vi "Write Alarms Event Response.vi"(8 "error in (no error)":errorcluster, 10 "Alarms":T1[](array[typedef]), 11 "Alarms in":refnum<class "HK Alarms.lvclass">) -> (0 "error out":errorcluster, 3 "Alarms out":refnum<class "HK Alarms.lvclass">)   [LabVIEW 2019, in "HK Alarms.lvclass"]
uses:
  HK Alarms/HK Alarms.lvclass
  HK Channel Settings Alarms.ctl
  HK Alarm enum Action.ctl
  HK Alarms/HK Alarms.lvclass/HK Alarms.ctl
  HK Item/HK Item.lvclass
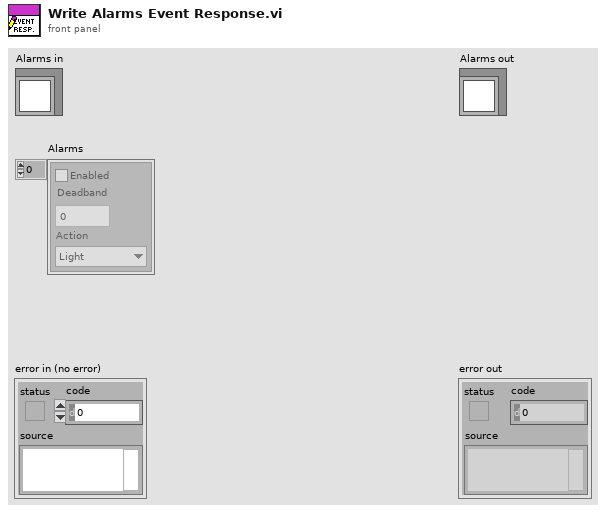
[diagram p1: front panel]
types:
  T1 = typedef "HK Item.lvclass/HK Channel Settings Alarms.ctl" = cluster{"Enabled":bool, "Deadband":i32, "Action":T2}
  T2 = typedef "HK Item.lvclass/HK Alarm enum Action.ctl" = enum16{"Light", "Message", "Safe"}
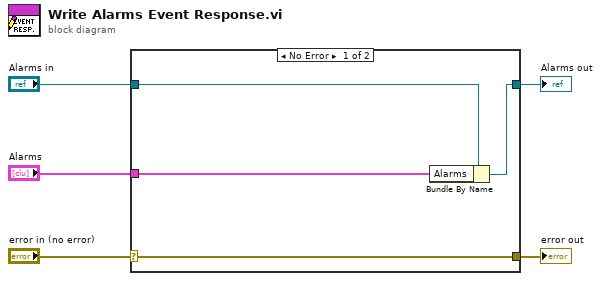
[diagram p0: block diagram]
diagram:
  n1 = case shown="No Error" "error in (no error)" {
    selector: "error in (no error)" -> [w9 w10]
    tunnel: [w9 w10] -> w4
    tunnel: [w7 w11] -> w2
    tunnel: "Alarms in" -> [w8 w11]
    tunnel: "Alarms" -> [w6 _]
    frame No Error {
      n2 = Bundle By Name(cluster=w8, "Alarms"=w6) -> (w7:refnum<class "HK Alarms.lvclass">)
    }
    frame Error {
    }
  }
  "error out" <- w4
  "Alarms out" <- w2
